vi "Joystick2_YAxis.vi"() -> ()   [LabVIEW 2016]
panel:
  out "Joystick2_YAxis":dbl
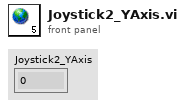
[diagram p1: front panel]
diagram:
